vi "Data File Processing UI.vi"() -> ()   [LabVIEW 2012]
doc: "This example shows how to create a built-in user interface (UI) in the Microphone Array Startup (MAS). You can create such a UI basing on the template named ma_analysis template.vi. Refer to <B>Example 3: Create a Simple UI</B> part in the Software Description of MAS for more information."
uses:
  sub VIs/Graph Tools.ctl
  sub VIs/Data File Processing UI Message Type Define.ctl
  sub VIs/Data File Processing UI_GlobalData.ctl
  sub VIs/Data File Processing UI Message Define.ctl
  sub VIs/FullFile.vi
panel:
  in  "Compute":bool
  in  "Graph Tool":T1
  in  "Return":bool
  in  "Save Project":bool
  in  "Open Project":bool
  out "Graph":waveform(dbl)[](graph)
  in  "Data List":string(tree)
  in  "Property Tab":enum32{"通道", "统计"}(tab)
  in  "TDMs Property":i32(listbox)
  in  "Compute Result":i32(listbox)
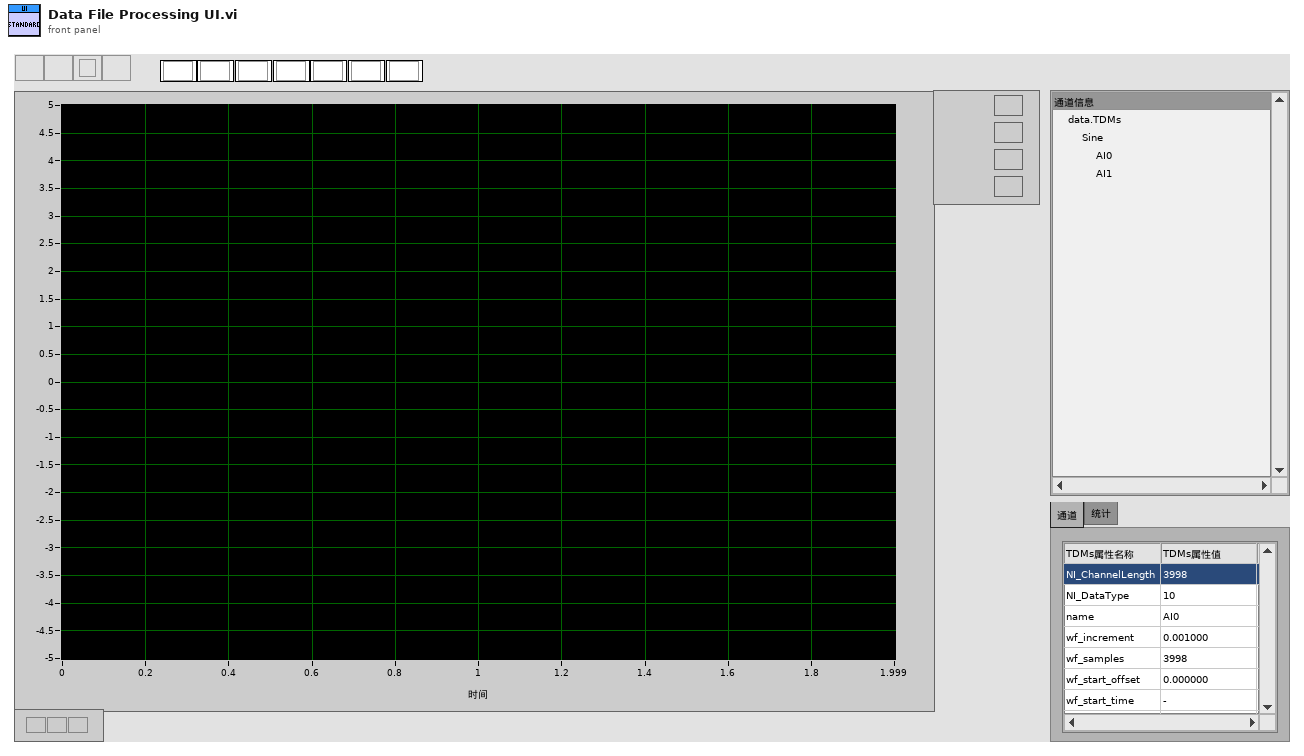
[diagram p1: front panel]
types:
  T1 = typedef "Graph Tools.ctl" = cluster{"Scroll Right":bool, "Scroll Left":bool, "Full Scale":bool, "Jump Right":bool, "Jump Left":bool, "Magnify":bool, "Select Entire Display":bool}
  T2 = typedef "Data File Processing UI_GlobalData.ctl" = cluster{"error":errorcluster, "CurrentFilePath":path, "File Start Time":dbl, "File End Time":dbl, "tdms file out":refnum<k34>}
  T3 = typedef "Data File Processing UI Message Type Define.ctl" = enum32{"Initialize", "SleepThread", "ErrorHandler", "NoEvent", "PreExit", "Exit", "----Action----", "OpenFile", "ReadAllCompute", "SaveFile", "RedrawGraph", "SelectChannel"}
  T4 = typedef "Data File Processing UI Message Define.ctl" = cluster{"data":variant, "type":T3}
  T5 = enum16{"JumpLeft", "JumpRight", "ScrollLeft", "ScrollRight"}
  T6 = cluster{"wf_increment":cluster{"Label":string, "Value":dbl}, "wf_start_time":cluster{"Label":string, "Value":timestamp}, "NI_ChannelLength":cluster{"Label":string, "Value":dbl}}[]
  T7 = enum32{"invalid app kind", "Development System", "Run Time System", "Student Edition", "Embedded LabVIEW", "Evaluation", "Custom"}
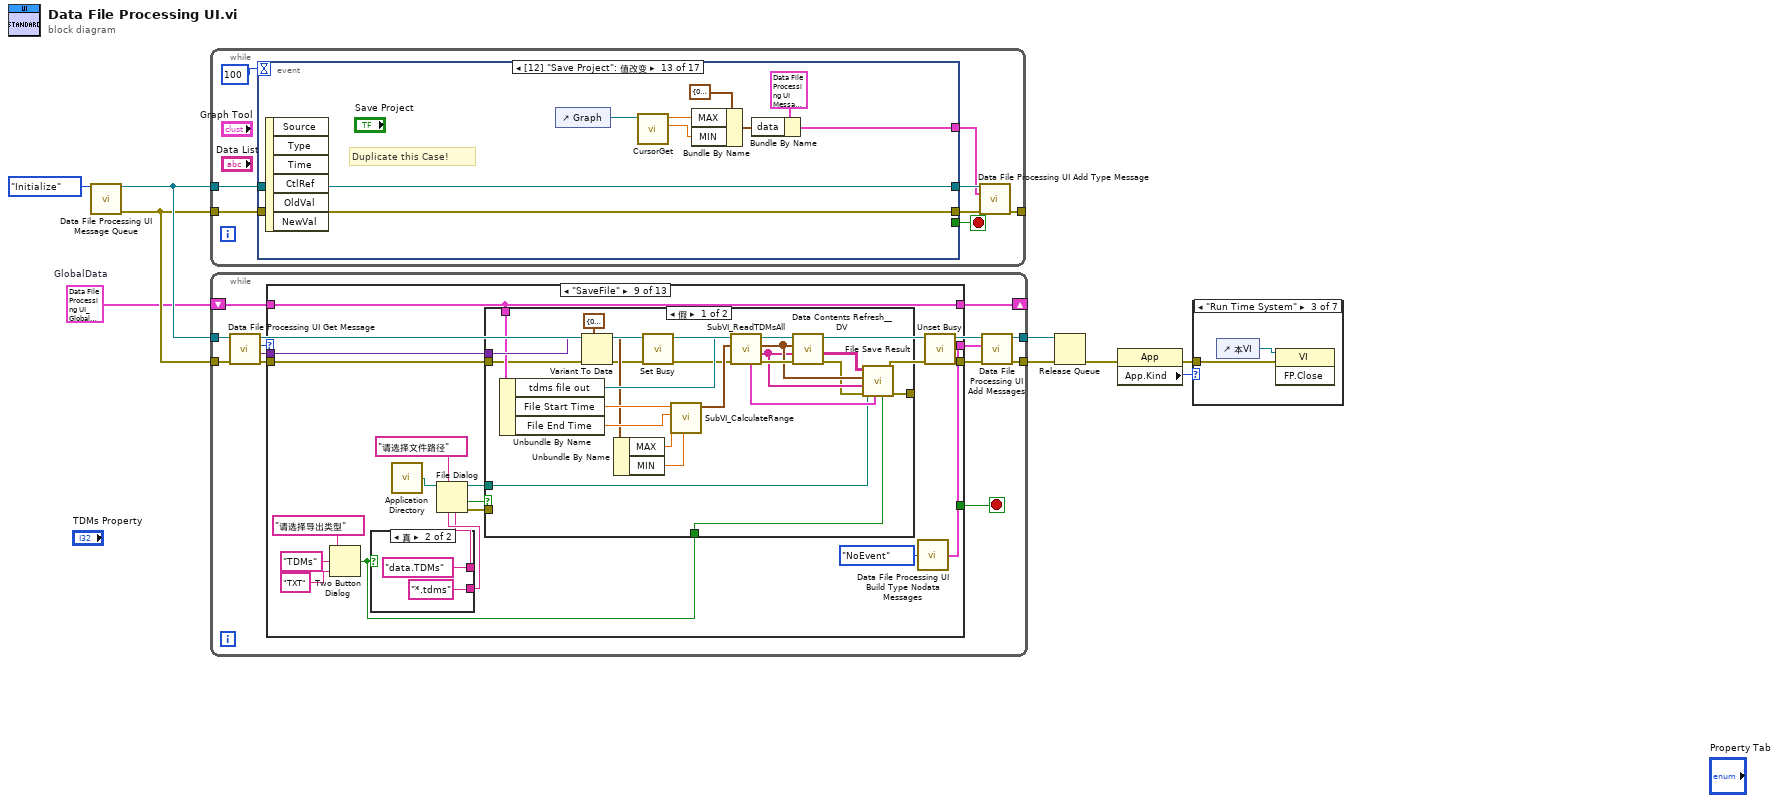
[diagram p0: block diagram]
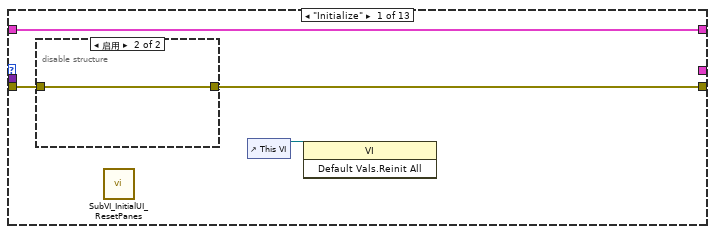
[diagram p8: hidden frame]
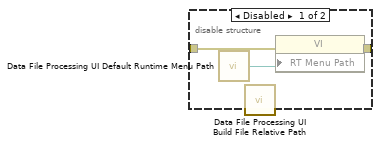
[diagram p9: hidden frame]
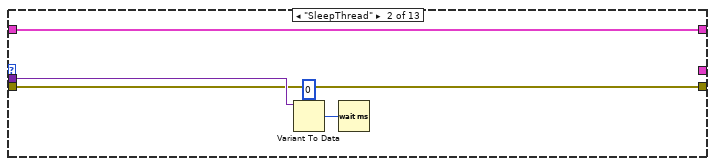
[diagram p10: hidden frame]
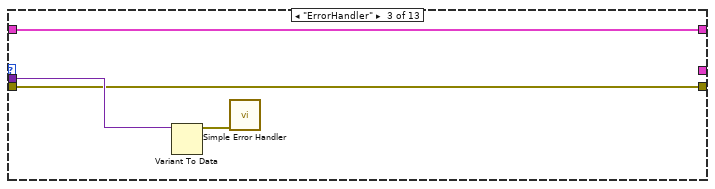
[diagram p11: hidden frame]
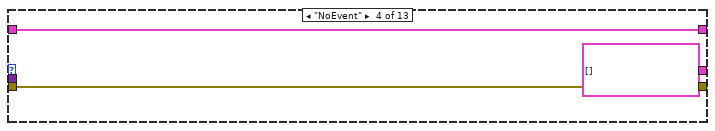
[diagram p12: hidden frame]
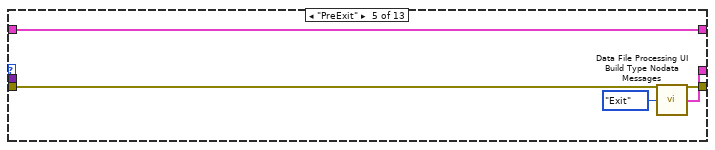
[diagram p13: hidden frame]
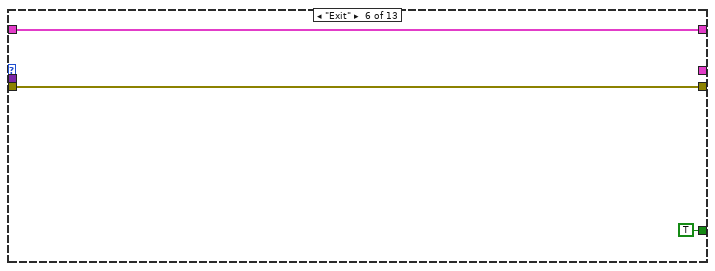
[diagram p14: hidden frame]
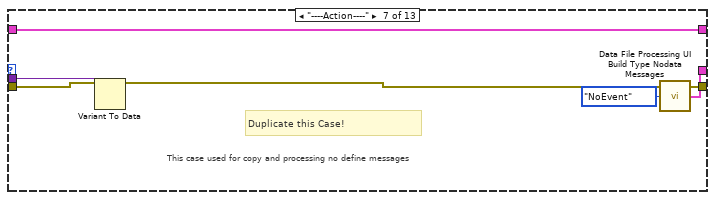
[diagram p15: hidden frame]
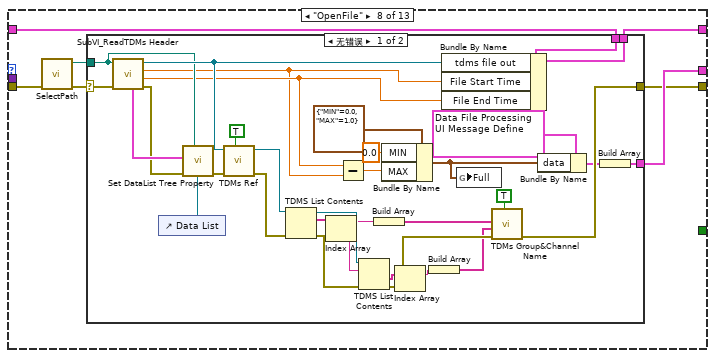
[diagram p16: hidden frame]
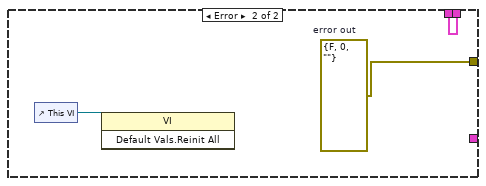
[diagram p17: hidden frame]
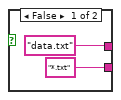
[diagram p18: hidden frame]
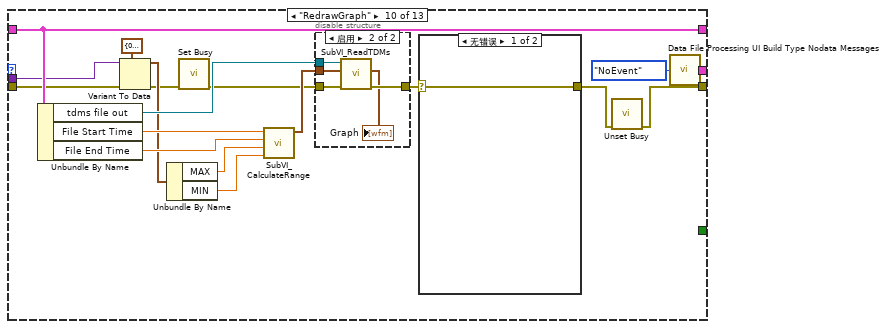
[diagram p20: hidden frame]
diagram:
  w5 = T2 {"error"={"status"=FALSE, "code"=0, "source"=""}, "CurrentFilePath"=path "", "File Start Time"=0.0, "File End Time"=0.0, "tdms file out"=refnum}  # GlobalData
  n1 = call "Data File Processing UI Message Queue.vi"("msg type"=Data_File_Processing_UI_Message_Type_Define."Initialize") -> ("queue out"=w8:refnum<queue>, "error out"=w7:errorcluster)  [unwired: 13 in]
  n2 = while {
    tunnel: w8 -> [w17]
    tunnel: w7 -> [w16]
    tunnel: [w12] -> _
    stop <- w15 stop-if-true
    n3 = event shown="[12] \"Save Project\": 值改变" {
      selector: _ -> [_ _ _ _ _ _ _ _ _ _ _ _ _ _ _ _ _]
      dyn-events: _ -> [_ _ _ _ _ _ _ _ _ _ _ _ _ _ _ _ _]
      timeout: 100 -> [_ _ _ _ _ _ _ _ _ _ _ _ _ _ _ _ _]
      tunnel: w17 -> [w21 w31 w65 w75 w81 w87 w93 w99 w105 w112 w118 w122 w131 w135 w138 w151 w159]
      tunnel: [w21 w31 w65 w75 w81 w87 w93 w99 w105 w112 w115 w122 w131 w135 w138 w151 w159] -> w14
      tunnel: w16 -> [w20 w27 w57 w70 w77 w83 w89 w95 w102 w111 w114 w121 w130 w134 w141 w150 w158]
      tunnel: [w20 w26 w56 w69 w76 w82 w88 w94 w101 w111 w113 w121 w130 w134 w141 w150 w158] -> w13
      tunnel: [_ _ _ _ _ _ _ _ _ _ _ _ _ _ w137 TRUE TRUE] -> w15
      tunnel: [w18 w23 w58 w73 T4 {"data"=variant, "type"=enum."NoEvent"} ("msg out") T4 {"data"=variant, "type"=enum."NoEvent"} ("msg out") T4 {"data"=variant, "type"=enum."NoEvent"} ("msg out") T4 {"data"=variant, "type"=enum."NoEvent"} ("msg out") w106 w109 w116 w119 w123 w132 w136 w149 w156] -> w11
      event Timeout {
        # "Duplicate this Case!"
        n4 = event-data() -> ()  [unwired: 2 out]
        n5 = call "Data File Processing UI Build Type Nodata Message.vi"("type"=Data_File_Processing_UI_Message_Type_Define."NoEvent" ("Msg")) -> ("msg out"=w18:T4)  [unwired: 14 out]
      }
      event "Data List": Value Change {
        n6 = event-data() -> ("NewVal"=w28:string)  [unwired: 5 out]
        n7 = call "TDMs Ref.vi"() -> ("error out"=w22:errorcluster, "tdms file out"=w25:refnum<k34>)  [unwired: 10 in]
        n8 = call <vilib>:"getNamesFromPath.vi"("error in (no error)"=w22, "tree path"=w28) -> ("error out"=w24:errorcluster, "channel"=w29:string, "group"=w30:string)  [unwired: 3 out]
        n9 = case shown="无错误" w24 {
          selector: w24 -> [w38 _]
          tunnel: w30 -> [w53 _]
          tunnel: w29 -> [w52 _]
          tunnel: w27 -> [w51 w55]
          tunnel: [w50 w55] -> w26
          tunnel: w25 -> [w49 _]
          tunnel: [w35 T4 {"data"=variant, "type"=enum."NoEvent"} ("msg out")] -> w23
          tunnel: [w34 _] -> _
          frame No Error {
            n10 = TDMS Get Properties(8:w38, 9:w52, 10:w53, 11:w49) -> (0:w43:errorcluster, 1:w33:string, 2:w44:string, 3:w45:refnum<k34>, 4:w47:variant[], 6:w48:string[])  [unwired: 2 out]
            n11 = call <vilib>:"formatPropertyList.vi"("property names"=w48, "property values"=w47) -> ("strings"=w46:string[][])
            n12 = call "getChannelList Modify.vi"("error in (no error)"=w43, "channel names"=w33, "group name"=w44, "tdms file"=w45) -> ("error out"=w37:errorcluster, "channel names out"=w39:string[], "group names out"=w40:string[])  [unwired: 1 out]
            n13 = call "TDMs Group&Channel Name.vi"("Ini?"=TRUE, "error in (no error)"=w37, "Channel"=w39, "Group"=w40) -> ("error out"=w34:errorcluster)  [unwired: 5 in, 2 out]
            n14 = control-ref of="TDMs Property"() -> (w42:refnum<vi>)
            n15 = property on="属性节点" class="MCListbox (严格)"(reference=w42, error in=w51, "ItemNames"=w46) -> (error out=w50:errorcluster)  [unwired: 1 out]
            n16 = global read "FullFile.vi" "Full"() -> (w32:cluster{"FullMIN":dbl, "FullMAX":dbl})
            n17 = Bundle By Name(cluster=T4 {"data"=variant, "type"=enum."RedrawGraph"} ("msg out"), "data"=w32) -> (w35:T4)
          }
          frame Error {
          }
        }
      }
      event "Compute": Value Change {
        # "2，添加计算功能。"
        n18 = event-data() -> ()  [unwired: 2 out]
        n19 = control-ref of="Graph"() -> (w63:refnum<vi>)
        n20 = call "CursorGet.vi"("错误输入"=w57, "WG"=w63) -> ("错误输出"=w56:errorcluster, "MIN"=w61:dbl, "MAX"=w60:dbl)  [unwired: 7 in]
        n21 = Bundle By Name(cluster=cluster{"MIN":dbl, "MAX":dbl} {"MIN"=0.0, "MAX"=1.0}, "MAX"=w60, "MIN"=w61) -> (w59:cluster{"MIN":dbl, "MAX":dbl})
        n22 = Bundle By Name(cluster=T4 {"data"=variant, "type"=enum."ReadAllCompute"} ("msg out"), "data"=w59) -> (w58:T4)
      }
      event Value Change {
        n23 = event-data() -> ()  [unwired: 5 out]
        n24 = control-ref of="Graph"() -> (w72:refnum<vi>)
        n25 = call "CursorSet.vi"("错误输入"=w70, "WG"=w72) -> ("错误输出"=w69:errorcluster, "MIN"=w68:dbl, "MAX"=w67:dbl)  [unwired: 7 in]
        n26 = Bundle By Name(cluster=cluster{"MIN":dbl, "MAX":dbl} {"MIN"=0.0, "MAX"=1.0}, "MAX"=w67, "MIN"=w68) -> (w66:cluster{"MIN":dbl, "MAX":dbl})
        n27 = Bundle By Name(cluster=T4 {"data"=variant, "type"=enum."RedrawGraph"} ("msg out"), "data"=w66) -> (w73:T4)
      }
      event Value Change {
        n28 = event-data() -> ()  [unwired: 5 out]
        n29 = control-ref of="Graph"() -> (w80:refnum<vi>)
        n30 = call "CursorMoveSet.vi"("Enum"=T5."ScrollRight", "错误输入"=w77, "WG"=w80) -> ("错误输出"=w76:errorcluster)  [unwired: 8 in]
      }
      event Value Change {
        n31 = event-data() -> ()  [unwired: 5 out]
        n32 = control-ref of="Graph"() -> (w86:refnum<vi>)
        n33 = call "CursorMoveSet.vi"("Enum"=T5."ScrollLeft", "错误输入"=w83, "WG"=w86) -> ("错误输出"=w82:errorcluster)  [unwired: 8 in]
      }
      event Value Change {
        n34 = event-data() -> ()  [unwired: 5 out]
        n35 = control-ref of="Graph"() -> (w92:refnum<vi>)
        n36 = call "CursorMoveSet.vi"("Enum"=T5."JumpRight", "错误输入"=w89, "WG"=w92) -> ("错误输出"=w88:errorcluster)  [unwired: 8 in]
      }
      event Value Change {
        n37 = event-data() -> ()  [unwired: 5 out]
        n38 = control-ref of="Graph"() -> (w98:refnum<vi>)
        n39 = call "CursorMoveSet.vi"("Enum"=T5."JumpLeft", "错误输入"=w95, "WG"=w98) -> ("错误输出"=w94:errorcluster)  [unwired: 8 in]
      }
      event Value Change {
        n40 = event-data() -> ()  [unwired: 4 out]
        n41 = control-ref of="Graph"() -> (w103:refnum<vi>)
        n42 = call "CursorSet.vi"("错误输入"=w102, "WG"=w103) -> ("错误输出"=w101:errorcluster)  [unwired: 7 in, 2 out]
        n43 = global read "FullFile.vi" "Full"() -> (w100:cluster{"FullMIN":dbl, "FullMAX":dbl})
        n44 = Bundle By Name(cluster=T4 {"data"=variant, "type"=enum."RedrawGraph"} ("msg out"), "data"=w100, "type"=Data_File_Processing_UI_Message_Type_Define."NoEvent") -> (w106:T4)
      }
      event Value Change {
        n45 = event-data() -> ()  [unwired: 2 out]
        n46 = global read "FullFile.vi" "Full"() -> (w108:cluster{"FullMIN":dbl, "FullMAX":dbl})
        n47 = Bundle By Name(cluster=T4 {"data"=variant, "type"=enum."RedrawGraph"} ("msg out"), "data"=w108) -> (w109:T4)
      }
      event "Graph": Scale Range Change {
        # "Duplicate this Case!"
        n48 = event-data() -> ()  [unwired: 7 out]
        n49 = Flush Queue(queue=w118, error in (no error)=w114) -> (queue out=w115:refnum<queue>, error out=w113:errorcluster)  [unwired: 1 out]
        n50 = call "Data File Processing UI Build Type Nodata Message.vi"("type"=Data_File_Processing_UI_Message_Type_Define."RedrawGraph" ("Msg")) -> ("msg out"=w116:T4)  [unwired: 14 out]
      }
      event "Open Project": Value Change {
        # "Duplicate this Case!"
        n51 = event-data() -> ()  [unwired: 7 out]
        n52 = call "Data File Processing UI Build Type Nodata Message.vi"("type"=Data_File_Processing_UI_Message_Type_Define."OpenFile" ("Msg")) -> ("msg out"=w119:T4)  [unwired: 14 out]
      }
      event "Save Project": Value Change {
        # "Duplicate this Case!"
        n53 = event-data() -> ()  [unwired: 7 out]
        n54 = control-ref of="Graph"() -> (w128:refnum<vi>)
        n55 = call "CursorGet.vi"("WG"=w128) -> ("MIN"=w126:dbl, "MAX"=w125:dbl)  [unwired: 8 in, 1 out]
        n56 = Bundle By Name(cluster=cluster{"MIN":dbl, "MAX":dbl} {"MIN"=0.0, "MAX"=1.0}, "MAX"=w125, "MIN"=w126) -> (w124:cluster{"MIN":dbl, "MAX":dbl})
        n57 = Bundle By Name(cluster=T4 {"data"=variant, "type"=enum."SaveFile"} ("msg out"), "data"=w124) -> (w123:T4)
      }
      event Panel Resize {
        n58 = event-data() -> ()  [unwired: 8 out]
        n59 = call "Data File Processing UI Build Type Nodata Message.vi"("type"=Data_File_Processing_UI_Message_Type_Define."NoEvent" ("Msg")) -> ("msg out"=w132:T4)  [unwired: 14 out]
      }
      event Menu Selection (User) {
        n60 = event-data() -> ("ItemTag"=w140:string, "ItemPath"=w139:string)  [unwired: 1 out]
        n61 = case shown="\"EXIT\"" w140 {
          tunnel: w139 -> [_ _]
          tunnel: [_ TRUE] -> w137
          tunnel: [w143 w145] -> w136
          frame Default {
            # "Duplicate this Case!"
            n62 = call "Data File Processing UI Build Type Nodata Message.vi"("type"=Data_File_Processing_UI_Message_Type_Define."NoEvent" ("Msg")) -> ("msg out"=w143:T4)  [unwired: 14 out]
          }
          frame "EXIT" {
            n63 = call "Data File Processing UI Build Type Nodata Message.vi"("type"=Data_File_Processing_UI_Message_Type_Define."PreExit" ("Msg")) -> ("msg out"=w145:T4)  [unwired: 14 out]
          }
        }
      }
      event Panel Close? {
        n64 = event-data() -> ()  [unwired: 2 out]
        n65 = call "Data File Processing UI Build Type Nodata Message.vi"("type"=Data_File_Processing_UI_Message_Type_Define."PreExit" ("Msg")) -> ("msg out"=w149:T4)  [unwired: 14 out]
        n66 = event-data("Discard?"=TRUE) -> ()  [unwired: 1 in, 1 out]
      }
      event "Return": Value Change {
        n67 = event-data() -> ()  [unwired: 7 out]
        n68 = Not(x="Return") -> (.not. x?=w153:bool)
        n69 = property on="Return" class="Bool (严格)"("Value"=w153) -> ()  [unwired: 2 in, 2 out]
        n70 = call "Data File Processing UI Build Type Nodata Message.vi"("type"=Data_File_Processing_UI_Message_Type_Define."PreExit" ("Msg")) -> ("msg out"=w156:T4)  [unwired: 14 out]
      }
    }
    n71 = call "Data File Processing UI Add Type Message.vi"("queue in"=w14, "Msg"=w11, "error in"=w13) -> ("error out"=w12:errorcluster)  [unwired: 12 out]
  }
  n72 = while {
    shift-right: [w170] -> _
    shift-left: w5 -> [w171]
    tunnel: w8 -> [w165]
    tunnel: [w160] -> w9
    tunnel: w7 -> [w166]
    tunnel: [w164] -> w4
    stop <- w172 stop-if-true
    n73 = call "Data File Processing UI Get Message.vi"("error in"=w166, "msg queue in"=w165) -> ("error out"=w169:errorcluster, "data"=w168:variant, "msg"=w167:T3, "msg queue out"=w162:refnum<queue>)  [unwired: 6 out]
    n74 = case shown="\"SaveFile\"" w167 {
      tunnel: [_ _ _ _ _ TRUE _ _ _ _ _ _ _] -> w172
      tunnel: [w174 w184 w187 w192 w196 w198 w200 w207 w263 w292 w321 w343 w347] -> w163
      tunnel: w169 -> [w175 w184 w187 w192 w196 w198 w200 w206 w259 w300 w333 w343 w347]
      tunnel: w171 -> [w176 w183 w189 w191 w195 w197 w201 w210 w260 w306 w339 w344 w348]
      tunnel: [w176 w183 w189 w191 w195 w197 w201 w208 w260 w306 w339 w344 w348] -> w170
      tunnel: [_ _ _ T4[] [] ("msg out") w194 _ w203 w211 w264 w309 w342 w346 w350] -> w161
      tunnel: w168 -> [_ w185 w188 _ _ _ w204 _ w261 w299 w332 _ w351]
      frame "Initialize" {
        n75 = disable-structure shown="启用" {
          disable-tunnel: w175 -> [w178 w180]
          disable-tunnel: [w177 w180] -> w174
          frame Disabled {
            n76 = call "Data File Processing UI Default Runtime Menu Path.vi"() -> ("runtime menu path"=w179:path)  [unwired: 15 in]
            n77 = call "Data File Processing UI Build File Relative Path.vi"() -> ()  [unwired: 15 in, 1 out]
            n78 = property class="VI"(error in=w178, "RT Menu Path"=w179) -> (error out=w177:errorcluster)  [unwired: 1 in, 1 out]
          }
          frame Enabled {
          }
        }
        n79 = call "SubVI_InitialUI_ResetPanes.vi"() -> ()  [unwired: 12 in]
        n80 = control-ref of="This VI"() -> (w173:refnum<vi>)
        n81 = invoke class="VI" method="Default Vals.Reinit All"(reference=w173) -> ()  [unwired: 2 in, 3 out]
      }
      frame "SleepThread" {
        n82 = Variant To Data(type=u32 0 ("milliseconds to wait"), Variant=w185) -> (data=w181:u32)  [unwired: 1 in, 1 out]
        n83 = Wait (ms)(milliseconds to wait=w181) -> ()  [unwired: 1 out]
      }
      frame "ErrorHandler" {
        n84 = Variant To Data(Variant=w188) -> (data=w186:errorcluster)  [unwired: 2 in, 1 out]
        n85 = call <vilib>:"Simple Error Handler.vi"("error in (no error)"=w186) -> ()  [unwired: 1 in, 8 out]
      }
      frame "NoEvent" {
      }
      frame "PreExit" {
        n86 = call "Data File Processing UI Build Type Nodata Messages.vi"("type"=Data_File_Processing_UI_Message_Type_Define."Exit") -> ("msg out"=w194:T4[])  [unwired: 14 out]
      }
      frame "Exit" {
      }
      frame "----Action----" {
        # "Duplicate this Case!"
        # "This case used for copy and processing no define messages"
        n87 = Variant To Data(type=w200, Variant=w204) -> ()  [unwired: 1 in, 2 out]
        n88 = call "Data File Processing UI Build Type Nodata Messages.vi"("type"=Data_File_Processing_UI_Message_Type_Define."NoEvent") -> ("msg out"=w203:T4[])  [unwired: 14 in]
      }
      frame "OpenFile" {
        n89 = call "SelectPath.vi"("error in (no error)"=w206) -> ("error out"=w205:errorcluster, "selected path"=w209:path)  [unwired: 9 in]
        n90 = case shown="无错误" w205 {
          selector: w205 -> [w241 _]
          tunnel: [w218 _] -> w211
          tunnel: w210 -> [w243 w246]
          tunnel: w209 -> [w234 _]
          tunnel: [w242 w246] -> w208
          tunnel: [w221 w245] -> w207
          frame No Error {
            n91 = call "SubVI_ReadTDMs Header.vi"("error in"=w241, "file path (use dialog)"=w234) -> ("error out"=w239:errorcluster, "StopTime"=w214:dbl, "StartTime"=w213:dbl, "tdms file out"=w236:refnum<k34>, "Group&ChName"=w240:cluster{"Group":string, "ChName":string[]}[])  [unwired: 5 in]
            n92 = control-ref of="Data List"() -> (w238:refnum<vi>)
            n93 = call "Set DataList Tree Property.vi"("file path"=w234, "error in (no error)"=w239, "Group&ChName"=w240, "Tree Ref"=w238) -> ("error out"=w237:errorcluster)  [unwired: 6 in, 1 out]
            n94 = call "TDMs Ref.vi"("Ini?"=TRUE, "error in (no error)"=w237, "tdms file out"=w236) -> ("error out"=w231:errorcluster, "tdms file out"=w233:refnum<k34>)  [unwired: 7 in]
            n95 = TDMS List Contents(4:w231, 7:w233) -> (0:w228:errorcluster, 2:w232:string[], 3:w229:refnum<k34>)  [unwired: 1 in, 1 out]
            n96 = Index Array(array=w232) -> (element=w227:string)  [unwired: 1 in]
            n97 = Subtract(x=w214, y=w213) -> (x-y=w215:dbl)
            n98 = TDMS List Contents(4:w228, 6:w227, 7:w229) -> (0:w225:errorcluster, 1:w223:string[])  [unwired: 2 out]
            n99 = Build Array(w227) -> (w226:string[])
            n100 = Bundle By Name(cluster=cluster{"MIN":dbl, "MAX":dbl} {"MIN"=0.0, "MAX"=1.0}, "MIN"=0.0, "MAX"=w215) -> (w212:cluster{"MIN":dbl, "MAX":dbl})
            n101 = Index Array(array=w223) -> (element=w222:string)  [unwired: 1 in]
            n102 = Build Array(w222) -> (w224:string[])
            n103 = Bundle By Name(cluster=w243, "tdms file out"=w236, "File Start Time"=w213, "File End Time"=w214) -> (w242:T2)
            n104 = global write "FullFile.vi" "Full"(w212) -> ()
            n105 = call "TDMs Group&Channel Name.vi"("Ini?"=TRUE, "error in (no error)"=w225, "Channel"=w224, "Group"=w226) -> ("error out"=w221:errorcluster)  [unwired: 5 in, 2 out]
            n106 = Bundle By Name(cluster=T4 {"data"=variant, "type"=enum."RedrawGraph"} ("msg out"), "data"=w212) -> (w219:T4)
            n107 = Build Array(w219) -> (w218:T4[])
          }
          frame Error {
            w245 = errorcluster {"status"=FALSE, "code"=0, "source"=""}  # error out
            n108 = control-ref of="This VI"() -> (w244:refnum<vi>)
            n109 = invoke class="VI" method="Default Vals.Reinit All"(reference=w244) -> ()  [unwired: 2 in, 3 out]
          }
        }
      }
      frame "SaveFile" {
        n110 = Two Button Dialog(message="请选择导出类型" ("消息"), 1:"TXT" ("T按钮名称（“确定”）"), 2:"TDMs" ("T按钮名称（“确定”）")) -> (T button?=w247:bool)
        n111 = case shown="真" w247 {
          tunnel: ["data.txt" ("默认名称") "data.TDMs" ("默认名称")] -> w248
          tunnel: ["*.txt" ("类型（所有文件）") "*.tdms" ("类型（所有文件）")] -> w249
          frame False {
          }
          frame True {
          }
        }
        n112 = call <vilib>:"Application Directory.vi"() -> ("Application Directory"=w257:path)
        n113 = File Dialog(6:w249, 7:"请选择文件路径" ("提示"), 9:w248, 11:w257) -> (0:w254:errorcluster, 1:w255:bool, 3:w253:path)  [unwired: 3 in, 1 out]
        n114 = case shown="假" w255 {
          tunnel: w261 -> [w282 _]
          tunnel: w260 -> [w281 _]
          tunnel: w259 -> [w280 w291]
          tunnel: [w272 w291] -> w258
          tunnel: w254 -> [_ _]
          tunnel: w253 -> [w270 _]
          tunnel: w247 -> [w269 _]
          frame False {
            n115 = Unbundle By Name(w281) -> ("tdms file out"=w287:refnum<k34>, "File Start Time"=w290:dbl, "File End Time"=w289:dbl)
            n116 = Variant To Data(error in=w280, type=cluster{"MIN":dbl, "MAX":dbl} {"MIN"=0.0, "MAX"=1.0}, Variant=w282) -> (data=w285:cluster{"MIN":dbl, "MAX":dbl}, error out=w279:errorcluster)
            n117 = Unbundle By Name(w285) -> ("MAX"=w284:dbl, "MIN"=w283:dbl)
            n118 = call <vilib>:"Set Busy.vi"("error in (no error)"=w279) -> ("error out"=w278:errorcluster)  [unwired: 9 in, 1 out]
            n119 = call "SubVI_CalculateRange.vi"("XScale.Minimum"=w283, "XScale.Maximum"=w284, "File End Time"=w289, "File Start Time"=w290) -> ("Range"=w288:cluster{dbl, dbl})  [unwired: 7 in]
            n120 = call "SubVI_ReadTDMsAll.vi"("error in"=w278, "Range Slide"=w288, "tdms文件输出"=w287) -> ("error out"=w277:errorcluster, "wfm name"=w274:string[], "WFM Out"=w275:waveform(dbl)[], "wfm Info"=w271:T6)  [unwired: 4 in, 1 out]
            n121 = call "Data Contents Refresh__DV.vi"("error in"=w277, "Wfm Name"=w274, "Graph Refreshed"=w275) -> ("error out"=w273:errorcluster, "Compute Result"=w276:string[][])  [unwired: 7 in]
            n122 = call "File Save Result.vi"("TDMs?"=w269, "wfm Info"=w271, "file path"=w270, "error in"=w273, "wfm name"=w274, "WFM Out"=w275, "Compute Result"=w276) -> ("error out"=w272:errorcluster)  [unwired: 4 in]
          }
          frame True {
          }
        }
        n123 = call "Data File Processing UI Build Type Nodata Messages.vi"("type"=Data_File_Processing_UI_Message_Type_Define."NoEvent") -> ("msg out"=w264:T4[])  [unwired: 14 in]
        n124 = call <vilib>:"Unset Busy.vi"("error in (no error)"=w258) -> ("error out"=w263:errorcluster)  [unwired: 10 in]
      }
      frame "RedrawGraph" {
        n125 = Unbundle By Name(w306) -> ("tdms file out"=w302:refnum<k34>, "File Start Time"=w305:dbl, "File End Time"=w304:dbl)
        n126 = Variant To Data(error in=w300, type=cluster{"MIN":dbl, "MAX":dbl} {"MIN"=0.0, "MAX"=1.0}, Variant=w299) -> (data=w298:cluster{"MIN":dbl, "MAX":dbl}, error out=w295:errorcluster)
        n127 = Unbundle By Name(w298) -> ("MAX"=w297:dbl, "MIN"=w296:dbl)
        n128 = call <vilib>:"Set Busy.vi"("error in (no error)"=w295) -> ("error out"=w294:errorcluster)  [unwired: 9 in, 1 out]
        n129 = call "SubVI_CalculateRange.vi"("XScale.Minimum"=w296, "XScale.Maximum"=w297, "File End Time"=w304, "File Start Time"=w305) -> ("Range"=w303:cluster{dbl, dbl})  [unwired: 7 in]
        n130 = disable-structure shown="启用" {
          disable-tunnel: w294 -> [w313 w317]
          disable-tunnel: [w312 w316] -> w308
          disable-tunnel: w302 -> [w311 w318]
          disable-tunnel: w303 -> [w310 w315]
          frame Disabled {
            n131 = call "SubVI_ReadTDMs.vi"("error in"=w313, "Range Slide"=w310, "tdms文件输出"=w311) -> ("error out"=w312:errorcluster)  [unwired: 6 in, 2 out]
          }
          frame Enabled {
            n132 = call "SubVI_ReadTDMs.vi"("error in"=w317, "Range Slide"=w315, "tdms文件输出"=w318) -> ("error out"=w316:errorcluster, "WFM Out"=→"Graph":waveform(dbl)[])  [unwired: 6 in, 1 out]
          }
        }
        n133 = case shown="无错误" w308 {
          selector: w308 -> [w319 _]
          tunnel: [w319 w320] -> w293
          frame No Error {
          }
          frame Error {
            w320 = errorcluster {"status"=FALSE, "code"=0, "source"=""}  # error IO
          }
        }
        n134 = call <vilib>:"Unset Busy.vi"("error in (no error)"=w293) -> ("error out"=w292:errorcluster)  [unwired: 10 in]
        n135 = call "Data File Processing UI Build Type Nodata Messages.vi"("type"=Data_File_Processing_UI_Message_Type_Define."NoEvent") -> ("msg out"=w309:T4[])  [unwired: 14 in]
      }
      frame "ReadAllCompute" {
        n136 = Unbundle By Name(w339) -> ("tdms file out"=w335:refnum<k34>, "File Start Time"=w338:dbl, "File End Time"=w337:dbl)
        n137 = Variant To Data(error in=w333, type=cluster{"MIN":dbl, "MAX":dbl} {"MIN"=0.0, "MAX"=1.0}, Variant=w332) -> (data=w331:cluster{"MIN":dbl, "MAX":dbl}, error out=w324:errorcluster)
        n138 = Unbundle By Name(w331) -> ("MAX"=w330:dbl, "MIN"=w329:dbl)
        n139 = call <vilib>:"Set Busy.vi"("error in (no error)"=w324) -> ("error out"=w323:errorcluster)  [unwired: 9 in, 1 out]
        n140 = call "SubVI_CalculateRange.vi"("XScale.Minimum"=w329, "XScale.Maximum"=w330, "File End Time"=w337, "File Start Time"=w338) -> ("Range"=w336:cluster{dbl, dbl})  [unwired: 7 in]
        n141 = call "SubVI_ReadTDMsAll.vi"("error in"=w323, "Range Slide"=w336, "tdms文件输出"=w335) -> ("error out"=w341:errorcluster, "wfm name"=w327:string[], "WFM Out"=w328:waveform(dbl)[])  [unwired: 4 in, 2 out]
        n142 = call "Data Contents Refresh__DV.vi"("error in"=w341, "Wfm Name"=w327, "Graph Refreshed"=w328) -> ("error out"=w326:errorcluster, "Compute Result"=w325:string[][])  [unwired: 7 in]
        n143 = property on="Compute Result" class="MCListbox (严格)"(error in=w326, "ItemNames"=w325) -> (error out=w322:errorcluster)  [unwired: 1 in, 1 out]
        n144 = call <vilib>:"Unset Busy.vi"("error in (no error)"=w322) -> ("error out"=w321:errorcluster)  [unwired: 10 in]
        n145 = call "Data File Processing UI Build Type Nodata Messages.vi"("type"=Data_File_Processing_UI_Message_Type_Define."NoEvent") -> ("msg out"=w342:T4[])  [unwired: 14 in]
      }
      frame "SelectChannel" {
        n146 = call "Data File Processing UI Build Type Nodata Messages.vi"("type"=Data_File_Processing_UI_Message_Type_Define."NoEvent") -> ("msg out"=w346:T4[])  [unwired: 14 in]
      }
      frame Default {
        # "Duplicate this Case!"
        # "This case used for copy and processing no define messages"
        n147 = Variant To Data(type=w347, Variant=w351) -> ()  [unwired: 1 in, 2 out]
        n148 = call "Data File Processing UI Build Type Nodata Messages.vi"("type"=Data_File_Processing_UI_Message_Type_Define."NoEvent") -> ("msg out"=w350:T4[])  [unwired: 14 in]
      }
    }
    n149 = call "Data File Processing UI Add Messages.vi"("error in"=w163, "messages"=w161, "msg queue in"=w162) -> ("error out"=w164:errorcluster, "msg queue out"=w160:refnum<queue>)  [unwired: 7 out]
  }
  n150 = Release Queue(queue=w9, error in (no error)=w4) -> (error out=w2:errorcluster)  [unwired: 3 out]
  n151 = property class="App"(error in=w2) -> (error out=w1:errorcluster, "App.Kind"=w3:T7)  [unwired: 1 in, 1 out]
  n152 = case shown="\"Run Time System\"" w3 {
    tunnel: w1 -> [_ _ w352 _ _ _ _]
    frame "invalid app kind", Default {
    }
    frame "Development System" {
    }
    frame "Run Time System" {
      n153 = control-ref of="本VI"() -> (w353:refnum<vi>)
      n154 = invoke class="VI" method="FP.Close"(reference=w353, error in=w352) -> ()  [unwired: 1 in, 3 out]
    }
    frame "Student Edition" {
    }
    frame "Embedded LabVIEW" {
    }
    frame "Evaluation" {
    }
    frame "Custom" {
    }
  }
